vi "Main.vi"() -> ()   [LabVIEW 2015]
doc: "The myRIO Project template acquires acceleration data from the onboard accelerometer and displays the changes of acceleration values in a waveform chart."
panel:
  out "Changed array":dbl[][](array[numeric])
  out "first array":dbl[][](array[numeric])
  out "text 2":string
  in  "format string":string
  out "text":string
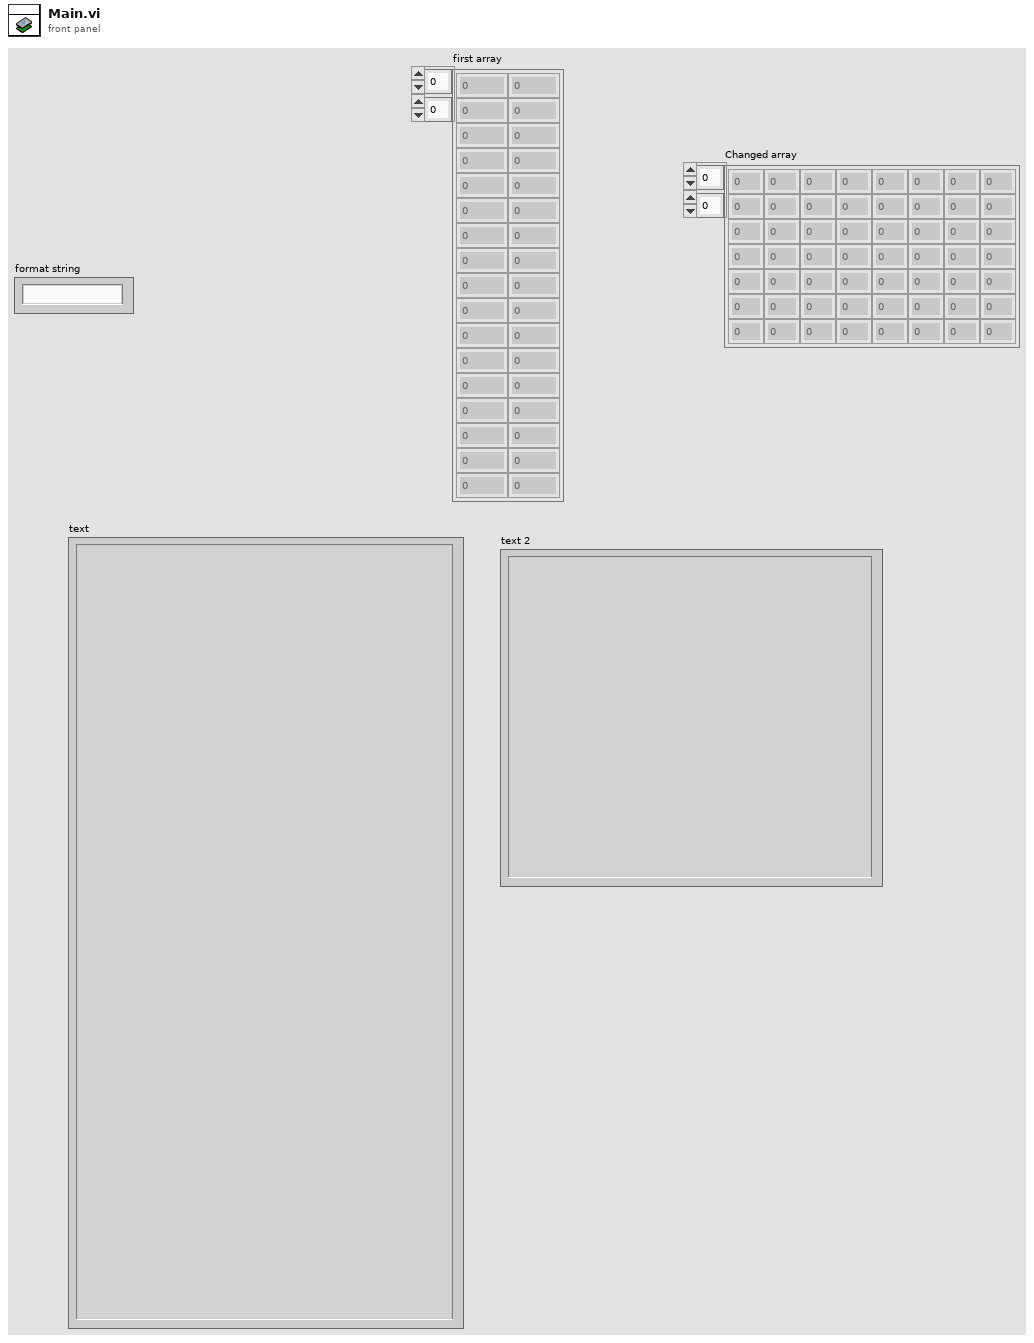
[diagram p1: front panel]
types:
  T1 = enum16{"open", "replace", "create", "open or create", "replace or create", "replace or create with confirmation"}
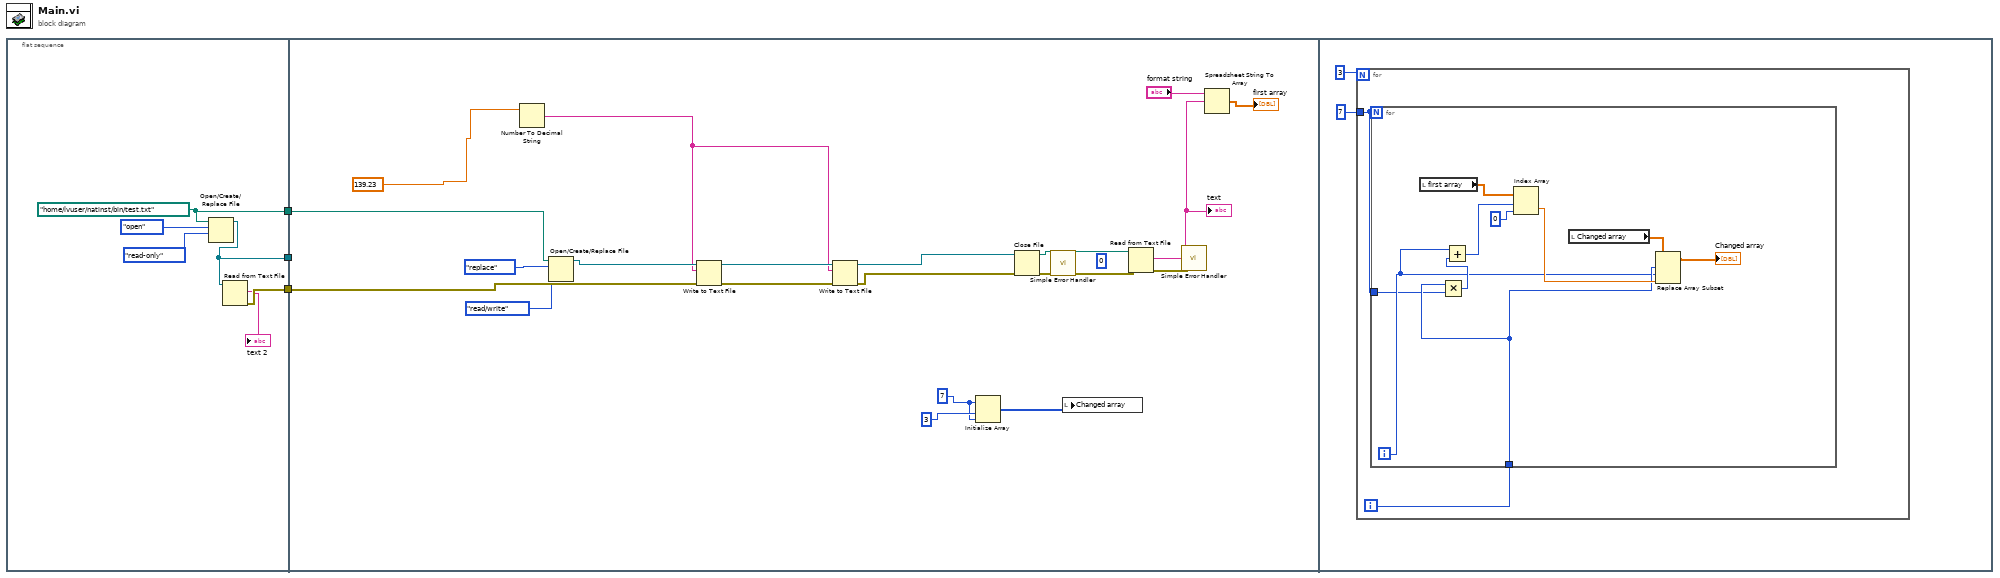
[diagram p0: block diagram]
diagram:
  n1 = flat-sequence {
    tunnel: [w8] -> w3
    tunnel: [w7] -> w2
    tunnel: [w5] -> w1
    tunnel: w3 -> [w24]
    tunnel: w2 -> [_]
    tunnel: w1 -> [w18]
    frame #0 {
      w5 = path "/home/lvuser/natinst/bin/test.txt" ("file path (use dialog)")
      n2 = Open/Create/Replace File(file path (use dialog)=w5, operation (0:open)=T1."open", access (0:read/write)=enum16{"read/write", "read-only", "write-only"}."read-only") -> (refnum out=w7:refnum<file>)  [unwired: 3 in, 2 out]
      n3 = Read from Text File(file (use dialog)=w7) -> (text=→"text 2":string, error out=w8:errorcluster)  [unwired: 3 in, 2 out]
    }
    frame #1 {
      w20 = 7
      (unwired) 0
      n4 = Number To Decimal String(number=139.23) -> (decimal integer string=w10:string)  [unwired: 1 in]
      n5 = Open/Create/Replace File(file path (use dialog)=w18, operation (0:open)=T1."replace", access (0:read/write)=enum16{"read/write", "read-only", "write-only"}."read/write") -> (refnum out=w19:refnum<file>)  [unwired: 3 in, 2 out]
      n6 = Write to Text File(file (use dialog)=w19, text=w10, error in=w24) -> (refnum out=w13:refnum<file>, error out=w14:errorcluster)  [unwired: 1 in, 1 out]
      n7 = Write to Text File(file (use dialog)=w13, text=w10, error in=w14) -> (refnum out=w12:refnum<file>, error out=w11:errorcluster)  [unwired: 1 in, 1 out]
      n8 = Initialize Array(w20, 3, w20) -> (w22:i32[][])
      n9 = Close File(refnum=w12, error in=w11) -> (path=w29:path, error out=w30:errorcluster)
      n10 = call <vilib>:"Simple Error Handler.vi"("error in (no error)"=w30) -> ("error out"=w28:errorcluster)  [unwired: 4 in, 4 out]
      n11 = local write "Changed array"(w22) -> ()
      n12 = Read from Text File(file (use dialog)=w29, error in=w28) -> (text=w26:string, error out=w27:errorcluster)  [unwired: 2 in, 2 out]
      "text" <- w26
      n13 = call <vilib>:"Simple Error Handler.vi"("error in (no error)"=w27) -> ()  [unwired: 4 in, 5 out]
      n14 = Spreadsheet String To Array(format string="format string", spreadsheet string=w26) -> (array=→"first array":dbl[][])  [unwired: 2 in]
    }
    frame #2 {
      n15 = for {
        N: 3 -> [_]
        tunnel: 7 -> [w33]
        i -> [w34]
        n16 = for {
          N: w33 -> [_]
          tunnel: w34 -> [w39]
          tunnel: w33 -> [w35]
          i -> [w36]
          n17 = local read "first array"() -> (w44:dbl[][])
          n18 = Multiply(x=w39, y=w35) -> (x*y=w38:i32)
          n19 = Add(x=w36, y=w38) -> (x+y=w37:i32)
          n20 = Index Array(array=w44, index (row)=w37, index (col)=0) -> (element=w41:dbl)
          n21 = local read "Changed array"() -> (w42:dbl[][])
          n22 = Replace Array Subset(array=w42, new element=w41, index (row)=w39, index (col)=w36) -> (→"Changed array":dbl[][])
        }
      }
    }
  }
